vi "Polar Plot - PG Circle.vi"(9 "grid measurements":T1 {"end angle" format="%0.2f"; "start angle" format="%0.2f"; "scale factors"."b" format="%0.2f"; "scale factors"."a" format="%0.2f"}, 10 "decade specs":cluster{"radius":i16, "label":string}[](array[cluster]), 11 "picture":picture) -> (3 "new picture":picture)   [LabVIEW 2020]
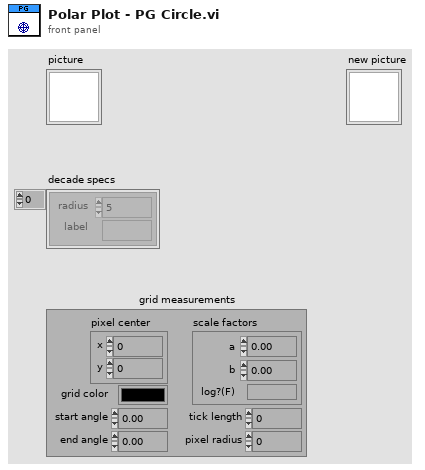
[diagram p1: front panel]
types:
  T1 = cluster{"pixel center":cluster{"x":i16, "y":i16}, "scale factors":cluster{"a":dbl, "b":dbl, "log?(F)":bool}, "grid color":u32, "start angle":dbl, "end angle":dbl, "tick length":i16, "pixel radius":i32}
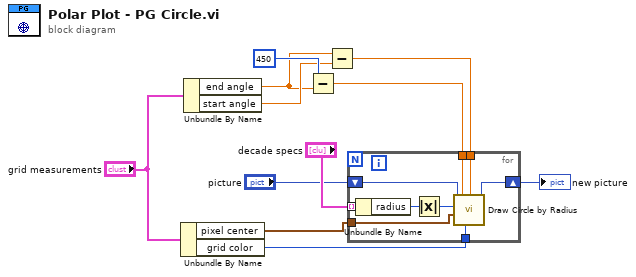
[diagram p0: block diagram]
diagram:
  n1 = Unbundle By Name("grid measurements") -> ("pixel center"=w9:cluster{"x":i16, "y":i16}, "grid color"=w10:u32)
  n2 = Unbundle By Name("grid measurements") -> ("end angle"=w2:dbl, "start angle"=w4:dbl)
  n3 = Subtract(x=450, y=w2) -> (x-y=w1:dbl)
  n4 = Subtract(x=w2, y=w4) -> (x-y=w3:dbl)
  n5 = for {
    tunnel: "decade specs" -> [w20] mode=indexing
    shift-right: [w17] -> w7
    shift-left: "picture" -> [w18]
    tunnel: w9 -> [w16]
    tunnel: w10 -> [w15]
    tunnel: w1 -> [w14]
    tunnel: w3 -> [w13]
    n6 = Unbundle By Name(w20) -> ("radius"=w19:i16)
    n7 = Absolute Value(x=w19) -> (abs(x)=w12:i16)
    n8 = call <vilib>:"Draw Circle by Radius.vi"("arc size(360)"=w13, "color(black)"=w15, "start angle(0)"=w14, "pixel center"=w16, "radius"=w12, "picture"=w18) -> ("new picture"=w17:picture)  [unwired: 5 in]
  }
  "new picture" <- w7
